vi "Particle Orientation Example.vi"() -> ()   [LabVIEW 2011]
doc: "This example shows how you can use particle analysis to determine the orientation of particles or objects in an image."
uses:
  <vilib>/vision/NI_Vision_Development_Module.lvlib
panel:
  out "Measurements":T1(plugin-control)
  out "Source":T1(plugin-control)
  out "Results":cluster{"X":sgl, "Y":sgl, "Angle":sgl}[](array[cluster]) {"Angle" format="%.1f"; "Y" format="%.1f"; "X" format="%.1f"}
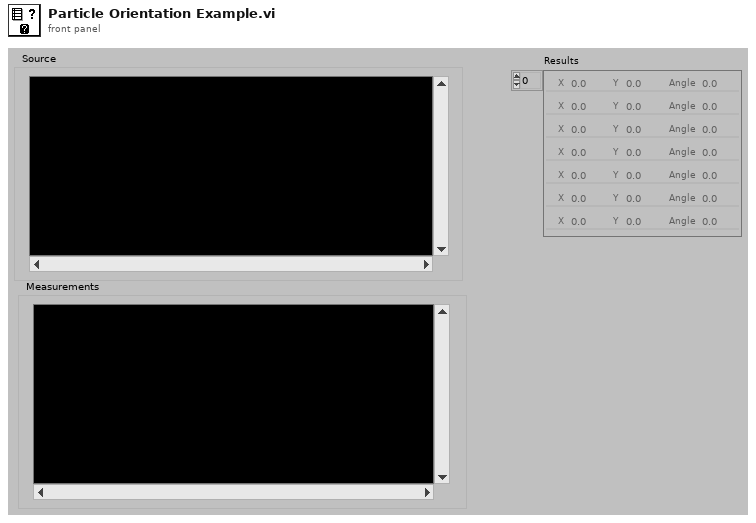
[diagram p1: front panel]
types:
  T1 = typedef "IMAQ Image.ctl" = refnum<image>
  T2 = typedef "Particle Parameters" = i32
  T3 = cluster{"Particle Measurements (Pixels)[0]":dbl, "Particle Measurements (Pixels)[1]":dbl, "Particle Measurements (Pixels)[2]":dbl}
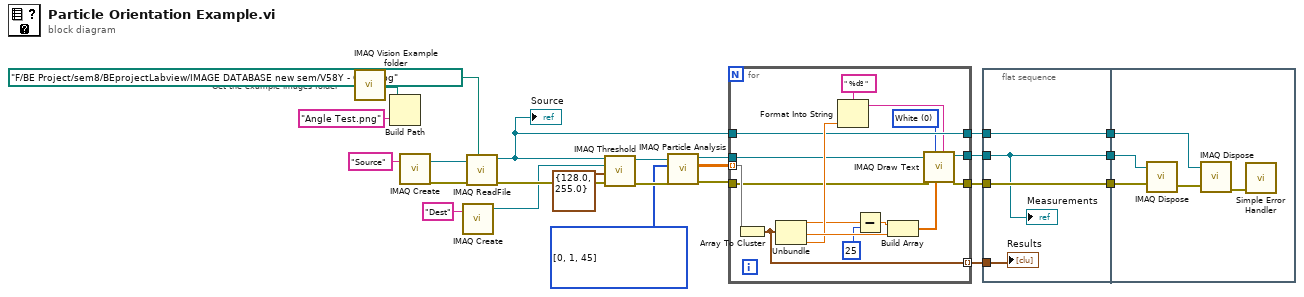
[diagram p0: block diagram]
diagram:
  w5 = T2[] [0, 1, 45] items=["Center of Mass X", "Center of Mass Y", "First Pixel X", "First Pixel Y", "Bounding Rect Left", "Bounding Rect Top", "Bounding Rect Right", "Bounding Rect Bottom", "Max Feret Diameter Start X", "Max Feret Diameter Start Y", "Max Feret Diameter End X", "Max Feret Diameter End Y", "Max Horiz. Segment Length Left", "Max Horiz. Segment Length Right", "Max Horiz. Segment Length Row", "-", "Bounding Rect Width", "Bounding Rect Height", "Bounding Rect Diagonal", "Perimeter", "Convex Hull Perimeter", "Holes' Perimeter", "Max Feret Diameter", "Equivalent Ellipse Major Axis", "Equivalent Ellipse Minor Axis", "Equivalent Ellipse Minor Axis (Feret)", "Equivalent Rect Long Side", "Equivalent Rect Short Side", "Equivalent Rect Diagonal", "Equivalent Rect Short Side (Feret)", "Average Horiz. Segment Length", "Average Vert. Segment Length", "Hydraulic Radius", "Waddel Disk Diameter", "-", "Area", "Holes' Area", "Particle & Holes' Area", "Convex Hull Area", "Image Area", "-", "Number of Holes", "Number of Horiz. Segments", "Number of Vert. Segments", "-", "Orientation", "Max Feret Diameter Orientation", "-", "% Area/Image Area", "% Area/(Particle & Holes' Area)", "Ratio of Equivalent Ellipse Axes", "Ratio of Equivalent Rect Sides", "-", "Elongation Factor", "Compactness Factor", "Heywood Circularity Factor", "Type Factor", "-", "Sum X", "Sum Y", "Sum XX", "Sum XY", "Sum YY", "Sum XXX", "Sum XXY", "Sum XYY", "Sum YYY", "-", "Moment of Inertia XX", "Moment of Inertia XY", "Moment of Inertia YY", "Moment of Inertia XXX", "Moment of Inertia XXY", "Moment of Inertia XYY", "Moment of Inertia YYY", "Norm. Moment of Inertia XX", "Norm. Moment of Inertia XY", "Norm. Moment of Inertia YY", "Norm. Moment of Inertia XXX", "Norm. Moment of Inertia XXY", "Norm. Moment of Inertia XYY", "Norm. Moment of Inertia YYY", "Hu Moment 1", "Hu Moment 2", "Hu Moment 3", "Hu Moment 4", "Hu Moment 5", "Hu Moment 6", "Hu Moment 7"] ("Pixel Measurements")
  # "Get the example images folder"
  n1 = call "IMAQ Vision Example folder.vi"() -> ("Example Image Path"=w24:path)  [unwired: 1 out]
  n2 = Build Path(base path=w24, name or relative path="Angle Test.png") -> ()  [unwired: 1 out]
  n3 = call "IMAQ Create"("Image Name"="Source") -> ("New Image"=w19:T1, "error out"=w18:errorcluster)  [unwired: 3 in, 1 out]
  n4 = call "IMAQ Create"("Image Name"="Dest") -> ("New Image"=w16:T1)  [unwired: 3 in, 2 out]
  n5 = call "IMAQ ReadFile"("File Path"=path "F:/BE Project/sem8/BEprojectLabview/IMAGE DATABASE new sem/V58Y - Copy.jpg", "error in (no error)"=w18, "Image"=w19) -> ("error out"=w17:errorcluster, "Image Out"=w14:T1)  [unwired: 2 in, 5 out]
  "Source" <- w14
  n6 = call "IMAQ Threshold"("error in (no error)"=w17, "Range"=cluster{"Lower value":sgl, "Upper value":sgl} {"Lower value"=128.0, "Upper value"=255.0}, "Image Dst"=w16, "Image Src"=w14) -> ("error out"=w6:errorcluster, "Image Dst Out"=w7:T1)  [unwired: 2 in, 4 out]
  n7 = call "IMAQ Particle Analysis"("error in (no error)"=w6, "Pixel Measurements"=w5, "Image"=w7) -> ("error out"=w4:errorcluster, "Particle Measurements (Pixels)"=w3:dbl[][], "Image Out (duplicate)"=w2:T1)  [unwired: 2 in, 4 out]
  n8 = for {
    tunnel: w3 -> [w38] mode=indexing
    tunnel: w4 -> [w30]
    tunnel: [w31] -> w15
    tunnel: w14 -> [w32]
    tunnel: [w32] -> w13
    tunnel: [w29] -> w10
    tunnel: [w28] -> w9 mode=indexing
    tunnel: w2 -> [w25]
    w26 = 0 items=["White", "Black", "Inverted", "Black on White", "White on Black"] ("Color")
    n9 = Array To Cluster(array=w38) -> (cluster=w28:T3)
    n10 = Unbundle(w28) -> ("Particle Measurements (Pixels)[0]"=w35:dbl, "Particle Measurements (Pixels)[1]"=w40:dbl, "Particle Measurements (Pixels)[2]"=w37:dbl)
    n11 = Format Into String(format string=" %dº ", w37) -> (resulting string=w27:string)  [unwired: 2 in, 1 out]
    n12 = Subtract(x=w35, y=25) -> (x-y=w33:dbl)
    n13 = Build Array(w33, w40) -> (w36:dbl[])
    n14 = call "IMAQ Draw Text"("String"=w27, "Insertion Point"=w36, "Color"=w26, "error in (no error)"=w30, "Image Src"=w25) -> ("error out"=w31:errorcluster, "Image Dst Out"=w29:T1)  [unwired: 2 in, 3 out]
  }
  n15 = flat-sequence {
    tunnel: w13 -> [w43]
    tunnel: w15 -> [w44]
    tunnel: [w44] -> w12
    tunnel: [w43] -> w11
    tunnel: w10 -> [w41]
    tunnel: w9 -> [w42]
    tunnel: [w41] -> w8
    tunnel: w12 -> [w49]
    tunnel: w11 -> [w45]
    tunnel: w8 -> [w46]
    frame #0 {
      "Results" <- w42
      "Measurements" <- w41
    }
    frame #1 {
      n16 = call "IMAQ Dispose"("Image"=w46, "error in (no error)"=w49) -> ("error out"=w48:errorcluster)  [unwired: 1 in, 3 out]
      n17 = call "IMAQ Dispose"("Image"=w45, "error in (no error)"=w48) -> ("error out"=w47:errorcluster)  [unwired: 1 in, 3 out]
      n18 = call <vilib>:"Simple Error Handler.vi"("error in (no error)"=w47) -> ()  [unwired: 1 in, 8 out]
    }
  }
